vi "Create Build Specification.vi"(8 "error in (no error)":errorcluster, 10 "Measurement Service Name":string, 11 "Project in":refnum<vi>) -> (0 "error out":errorcluster)   [LabVIEW 2020, in "MeasurementService Editor.lvlib"]
uses:
  MeasurementService Editor.lvlib
  <vilib>/AppBuilder/AB_API/common/AB_API Primary Exclusions.ctl
  <vilib>/AppBuilder/AB_Source_Property_WindowRunTimePosition.ctl
  NI_AB_API_EXE_Extensions/NI_AB_API_EXE_Extensions.lvclass
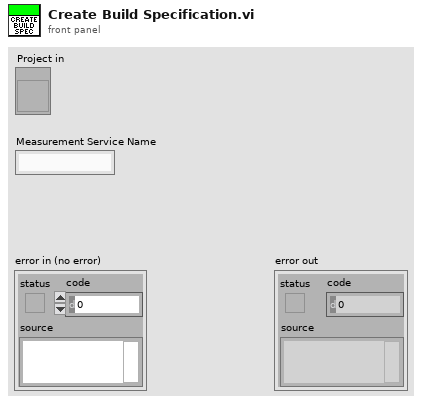
[diagram p1: front panel]
types:
  T1 = typedef "AB_Source_Property_WindowRunTimePosition.ctl" = enum16{"Unchanged", "Centered", "Maximized", "Minimized"}
  T2 = typedef "AB_API Primary Exclusions.ctl" = cluster{"Disconnect type definitions":bool, "Remove unused polymorphic VI instances":bool, "Remove unused members of project libraries":bool, "Modify project library file after removing unused members":bool}
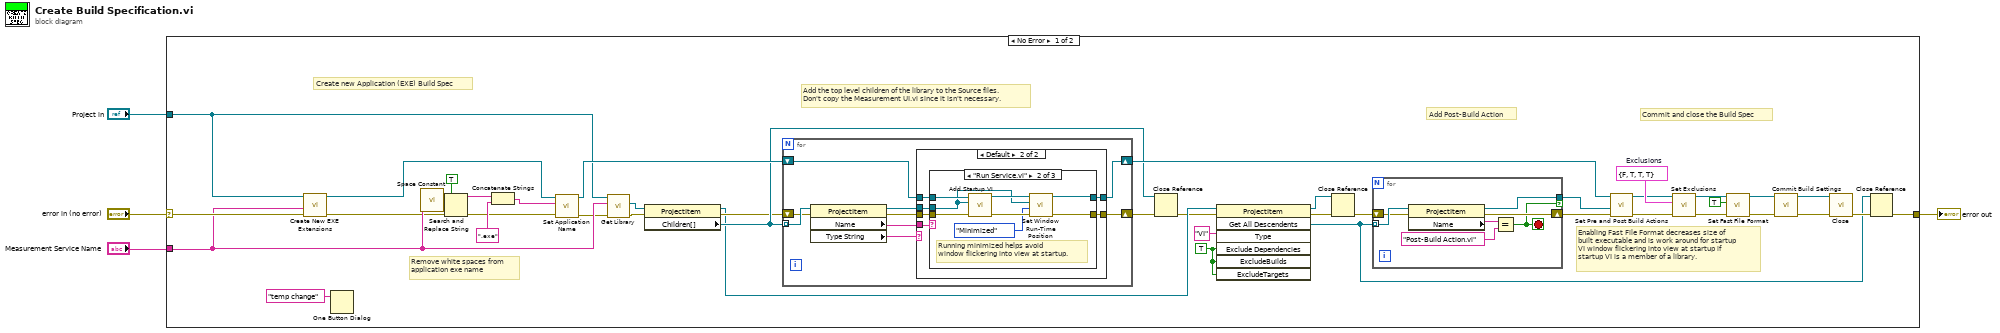
[diagram p0: block diagram]
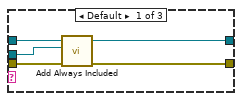
[diagram p3: hidden frame]
diagram:
  n1 = case shown="No Error" "error in (no error)" {
    selector: "error in (no error)" -> [w46 w86]
    tunnel: "Project in" -> [w22 _]
    tunnel: "Measurement Service Name" -> [w27 _]
    tunnel: [w17 w86] -> w3
    frame No Error {
      w30 = T2 {"Disconnect type definitions"=FALSE, "Remove unused polymorphic VI instances"=TRUE, "Remove unused members of project libraries"=TRUE, "Modify project library file after removing unused members"=TRUE}  # Exclusions
      w33 = TRUE ("ExcludeDependencies")
      # "Enabling Fast File Format decreases size of\nbuilt executable and is work around for startup\nVI window flickering into view at startup if\nstartup VI is a member of a library."
      # "Remove white spaces from application exe name"
      # "Create new Application (EXE) Build Spec"
      # "Commit and close the Build Spec"
      # "Add Post-Build Action"
      # "Add the top level children of the library to the Source files.\nDon't copy the Measurement UI.vi since it isn't necessary."
      n2 = call "Create New EXE Extensions.vi"("error in (no error)"=w46, "Build specification name"=w27, "Project Refnum"=w22) -> ("error out"=w11:errorcluster, "NI_AB_API_Build out"=w12:refnum<class "NI_AB_API_EXE_Extensions.lvclass">)  [unwired: 7 in]
      n3 = One Button Dialog(message="temp change") -> ()  [unwired: 1 in, 1 out]
      n4 = call <vilib>:"Space Constant.vi"() -> ("String"=w44:string)
      n5 = Search and Replace String(replace all?=TRUE ("replace all? (F)"), input string=w27, search string=w44, error in=w11) -> (result string=w43:string, error out=w38:errorcluster)  [unwired: 4 in, 2 out]
      n6 = Concatenate Strings(w43, ".exe" ("string")) -> (w41:string)
      n7 = call-dynamic "Set Application Name.vi"("error in (no error)"=w38, "Application file name"=w41, "EXE in"=w12) -> ("error out"=w24:errorcluster, "EXE out"=w40:refnum<class "NI_AB_API_EXE_Extensions.lvclass">)  [unwired: 7 in]
      n8 = call "Get Library.vi"("error in (no error)"=w24, "Library Name"=w27, "Project in"=w22) -> ("error out"=w26:errorcluster, "Library Item"=w25:refnum<vi>)  [unwired: 6 in, 1 out]
      n9 = property class="ProjectItem"(reference=w25, error in=w26) -> (reference out=w14:refnum<vi>, error out=w15:errorcluster, "Children[]"=w23:refnum<vi>[])
      n10 = for {
        tunnel: w23 -> [w62] mode=indexing
        shift-right: [w58] -> w39
        shift-left: w40 -> [w60]
        shift-right: [w55] -> w35
        shift-left: w15 -> [w57]
        n11 = property class="ProjectItem"(reference=w62, error in=w57) -> (reference out=w59:refnum<vi>, error out=w56:errorcluster, "Name"=w61:string, "Type String"=w54:string)
        n12 = case shown="Default" w54 {
          tunnel: w61 -> [_ w70]
          tunnel: w60 -> [w64 w69]
          tunnel: w59 -> [_ w68]
          tunnel: [w64 w67] -> w58
          tunnel: w56 -> [w63 w66]
          tunnel: [w63 w65] -> w55
          frame "Folder" {
          }
          frame Default {
            n13 = case shown="\"Run Service.vi\"" w70 {
              tunnel: w69 -> [w75 w83 w85]
              tunnel: w68 -> [w74 w77 _]
              tunnel: [w73 w80 w85] -> w67
              tunnel: w66 -> [w72 w82 w84]
              tunnel: [w71 w78 w84] -> w65
              frame Default {
                n14 = call-dynamic "Add Always Included.vi"("error in (no error)"=w72, "ProjectItem Refnum"=w74, "EXE in"=w75) -> ("error out"=w71:errorcluster, "EXE out"=w73:refnum<class "NI_AB_API_EXE_Extensions.lvclass">)  [unwired: 7 in]
              }
              frame "Run Service.vi" {
                # "Running minimized helps avoid\nwindow flickering into view at startup."
                n15 = call-dynamic "Add Startup VI.vi"("error in (no error)"=w82, "ProjectItem Refnum"=w77, "EXE in"=w83) -> ("error out"=w79:errorcluster, "EXE out"=w81:refnum<class "NI_AB_API_EXE_Extensions.lvclass">)  [unwired: 7 in]
                n16 = call "Set Window Run-Time Position.vi"("error in (no error)"=w79, "Window Run-Time Position"=AB_Source_Property_WindowRunTimePosition."Minimized", "ProjectItem Refnum"=w77, "NI_AB_API_EXE_Extensions in"=w81) -> ("error out"=w78:errorcluster, "NI_AB_API_EXE_Extensions out"=w80:refnum<class "NI_AB_API_EXE_Extensions.lvclass">)  [unwired: 6 in]
              }
              frame "Measurement UI.vi" {
              }
            }
          }
        }
      }
      n17 = Close Reference(reference=w23, error in (no error)=w35) -> (error out=w13:errorcluster)
      n18 = invoke class="ProjectItem" method="Get All Descendents"(reference=w14, error in=w13, "Type"="VI", "Exclude Dependencies"=w33, "ExcludeBuilds"=w33, "ExcludeTargets"=w33) -> (reference out=w21:refnum<vi>, error out=w20:errorcluster, "All Descendents"=w16:refnum<vi>[])  [unwired: 1 in, 4 out]
      n19 = Close Reference(reference=w21, error in (no error)=w20) -> (error out=w19:errorcluster)
      n20 = for {
        tunnel: w16 -> [w53] mode=indexing
        shift-right: [w50] -> w31
        shift-left: w19 -> [w48]
        tunnel: [w49] -> w32 if=w47
        stop <- w47 stop-if-true
        n21 = property class="ProjectItem"(reference=w53, error in=w48) -> (reference out=w49:refnum<vi>, error out=w50:errorcluster, "Name"=w51:string)
        n22 = Equal?(x=w51, y="Post-Build Action.vi") -> (x = y?=w47:bool)
      }
      n23 = call-dynamic "Set Pre and Post Build Actions.vi"("error in (no error)"=w31, "Post Build Action VI"=w32, "Build in"=w39) -> ("error out"=w28:errorcluster, "Build out"=w29:refnum<class "NI_AB_API_EXE_Extensions.lvclass">)  [unwired: 7 in]
      n24 = call-dynamic "Set Exclusions.vi"("error in (no error)"=w28, "Exclusions"=w30, "EXE in"=w29) -> ("error out"=w8:errorcluster, "EXE out"=w10:refnum<class "NI_AB_API_EXE_Extensions.lvclass">)  [unwired: 7 in]
      n25 = call "Set Fast File Format.vi"("error in (no error)"=w8, "Enable Fast File Format"=TRUE, "NI_AB_API_EXE_Extensions in"=w10) -> ("error out"=w7:errorcluster, "NI_AB_API_EXE_Extensions out"=w9:refnum<class "NI_AB_API_EXE_Extensions.lvclass">)  [unwired: 7 in]
      n26 = call-dynamic "Commit Build Settings.vi"("error in (no error)"=w7, "EXE in"=w9) -> ("error out"=w36:errorcluster, "EXE out"=w37:refnum<class "NI_AB_API_EXE_Extensions.lvclass">)  [unwired: 8 in]
      n27 = call-dynamic "Close.vi"("error in (no error)"=w36, "EXE in"=w37) -> ("error out"=w18:errorcluster)  [unwired: 9 in]
      n28 = Close Reference(reference=w16, error in (no error)=w18) -> (error out=w17:errorcluster)
    }
    frame Error {
    }
  }
  "error out" <- w3
